vi "FPGA Main.vi"() -> ()   [LabVIEW 2019]
uses:
  Program Files (x86)/National Instruments/LabVIEW 2019/examples/NI SPI IP/R Series/FPGA/Controls/R Series - SPI Master Control Signals.ctl
  <userlib>/_NI SPI IP/FPGA/Controllers/Public/Transfer Settings.ctl
  <vilib>/Platform/TimedLoop/XDataNode/timing_clust.ctl
  <vilib>/Platform/TimedLoop/XDataNode/nitl_modes.ctl
  <vilib>/Platform/TimedLoop/XDataNode/wakeup.ctl
  <userlib>/_NI SPI IP/FPGA/Controllers/Public/Spi Master Inputs.ctl
  <vilib>/rvi/Emulation/niFpgaGetClockAttributes.vi
  <vilib>/rvi/Emulation/niFpgaSctlEmulationGetInTimedLoop.vi
  <vilib>/rvi/Emulation/niFpgaEmulationReportErrorSimple.vi
  <vilib>/rvi/interface/RandomDataEmulation/nirviRandomDataMultiElementFPGAFIFO.vi
  <instcachedir>/0/nirviRandomDataMultiElementFPGAFIFO_1ED88BA00AC641F388A9B1FAA20E354D.lvgen/nirviRandomDataMultiElementFPGAFIFO_1ED88BA00AC641F388A9B1FAA20E354D_002.vi
  <vilib>/rvi/interface/RandomDataEmulation/niFpgaRandomDataHandleErrors.vi
  <vilib>/rvi/Memory/Memory_Emulation/nirvimemoryFastEmulation.vi
  <vilib>/rvi/Memory/Memory_Emulation/nirvimemoryEmulation.vi
  <vilib>/rvi/Emulation/niFpgaEmulationIsFPGAContextNoSignature.vi
  <vilib>/rvi/DataTransferAndStorage/Container/Common/niFpgaContainerGetUniqueNameForEmu.vi
  <vilib>/rvi/Emulation/niFpgaProcessEmulError.vi
  <vilib>/rvi/errors/nirviReportUnexpectedCaseInternalError (U32).vi
  <vilib>/rvi/Emulation/niFpgaCriticalErrorInLSC.vi
  <vilib>/rvi/eio/common/nirviEmuTemplateMethod_errors.vi
  <vilib>/rvi/DataTransferAndStorage/Container/XNode/niFpgaContainer.xnode
  <vilib>/rvi/interface/RandomDataEmulation/nirviRandomDataFpgaMultiElementTemplate.vi
  <vilib>/eio/EIONode/EIONode.xnode
  <vilib>/Platform/TimedLoop/XDataNode/XDataNode.xnode
  <vilib>/rvi/interface/RandomDataEmulation/nirviRandomDataFpgaReadWriteTemplate.vi
  <userlib>/_NI SPI IP/FPGA/Controllers/NI SPI IP FPGA.lvlib
  <vilib>/Platform/TimedLoop/XDataNode/XDNodeRunTimeDep.lvlib
panel:
  in  "Height":i32=320
  in  "Width":i32=480
  in  "StreamDisabled":bool=TRUE
  in  "Master Settings":T1
  out "Master Signals":T2
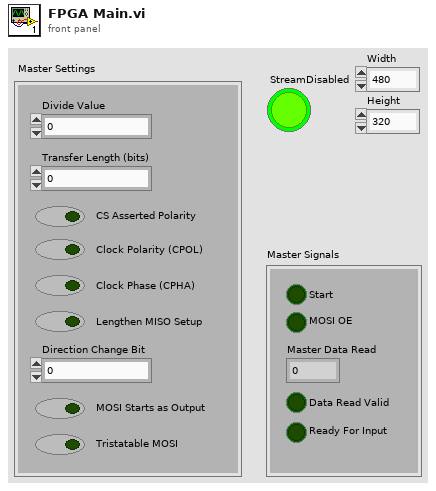
[diagram p1: front panel]
types:
  T1 = typedef "NI SPI IP FPGA.lvlib/Transfer Settings.ctl" = cluster{"Divide Value":u8, "Transfer Length (bits)":u8, "CS Asserted Polarity":bool, "Clock Polarity (CPOL)":bool, "Clock Phase (CPHA)":bool, "Lengthen MISO Setup":bool, "Direction Change Bit":u8, "MOSI Starts as Output":bool, "Tristatable MOSI":bool}
  T2 = typedef "R Series - SPI Master Control Signals.ctl" = cluster{"Start":bool, "MOSI OE":bool, "Master Data Read":u64, "Data Read Valid":bool, "Ready For Input":bool}
  T3 = typedef "XDNodeRunTimeDep.lvlib/timing_clust.ctl" = cluster{"Expected End [f-1]":u64, "Actual End [f-1]":u64, "Finished Late? [f-1]":bool, "Expected End [i-1]":u64, "Actual End [i-1]":u64, "Finished Late? [i-1]":bool, "Expected Start [i]":u64, "Actual Start [i]":u64, "Expected Start [f]":u64, "Actual Start [f]":u64, "Source Name":string, "Structure Name":string, "Period":i64, "Deadline":i64, "Offset":i64, "Start":i64, "Priority":i32, "Timeout":i32, "Mode":T4, "Wakeup Reason":T5, "Error":errorcluster, "Source Type":string, "Secondary Source Type":string, "Global End Time":u64, "Global Start Time":u64, "Frame Duration":u64, "Iteration Duration":u64, "Assigned CPU":i32, "I/O Scan Engine Mode":u32}
  T4 = typedef "XDNodeRunTimeDep.lvlib/nitl_modes.ctl" = enum32{"No Change", "Process missed periods, maintain original phase", "Discard missed periods, maintain original phase", "Process missed periods, ignore original phase", "Discard missed periods, ignore original phase"}
  T5 = typedef "XDNodeRunTimeDep.lvlib/wakeup.ctl" = enum32{"Normal", "Aborted", "Asynchronous wakeup", "Timing source error", "Timed loop error", "Timeout"}
  T6 = typedef "NI SPI IP FPGA.lvlib/Spi Master Inputs.ctl" = cluster{"MISO":bool}
  T7 = typedef "NI SPI IP FPGA.lvlib/Spi Master Outputs.ctl" = cluster{"Chip Select":bool, "Clock":bool, "MOSI":bool, "MOSI OE":bool}
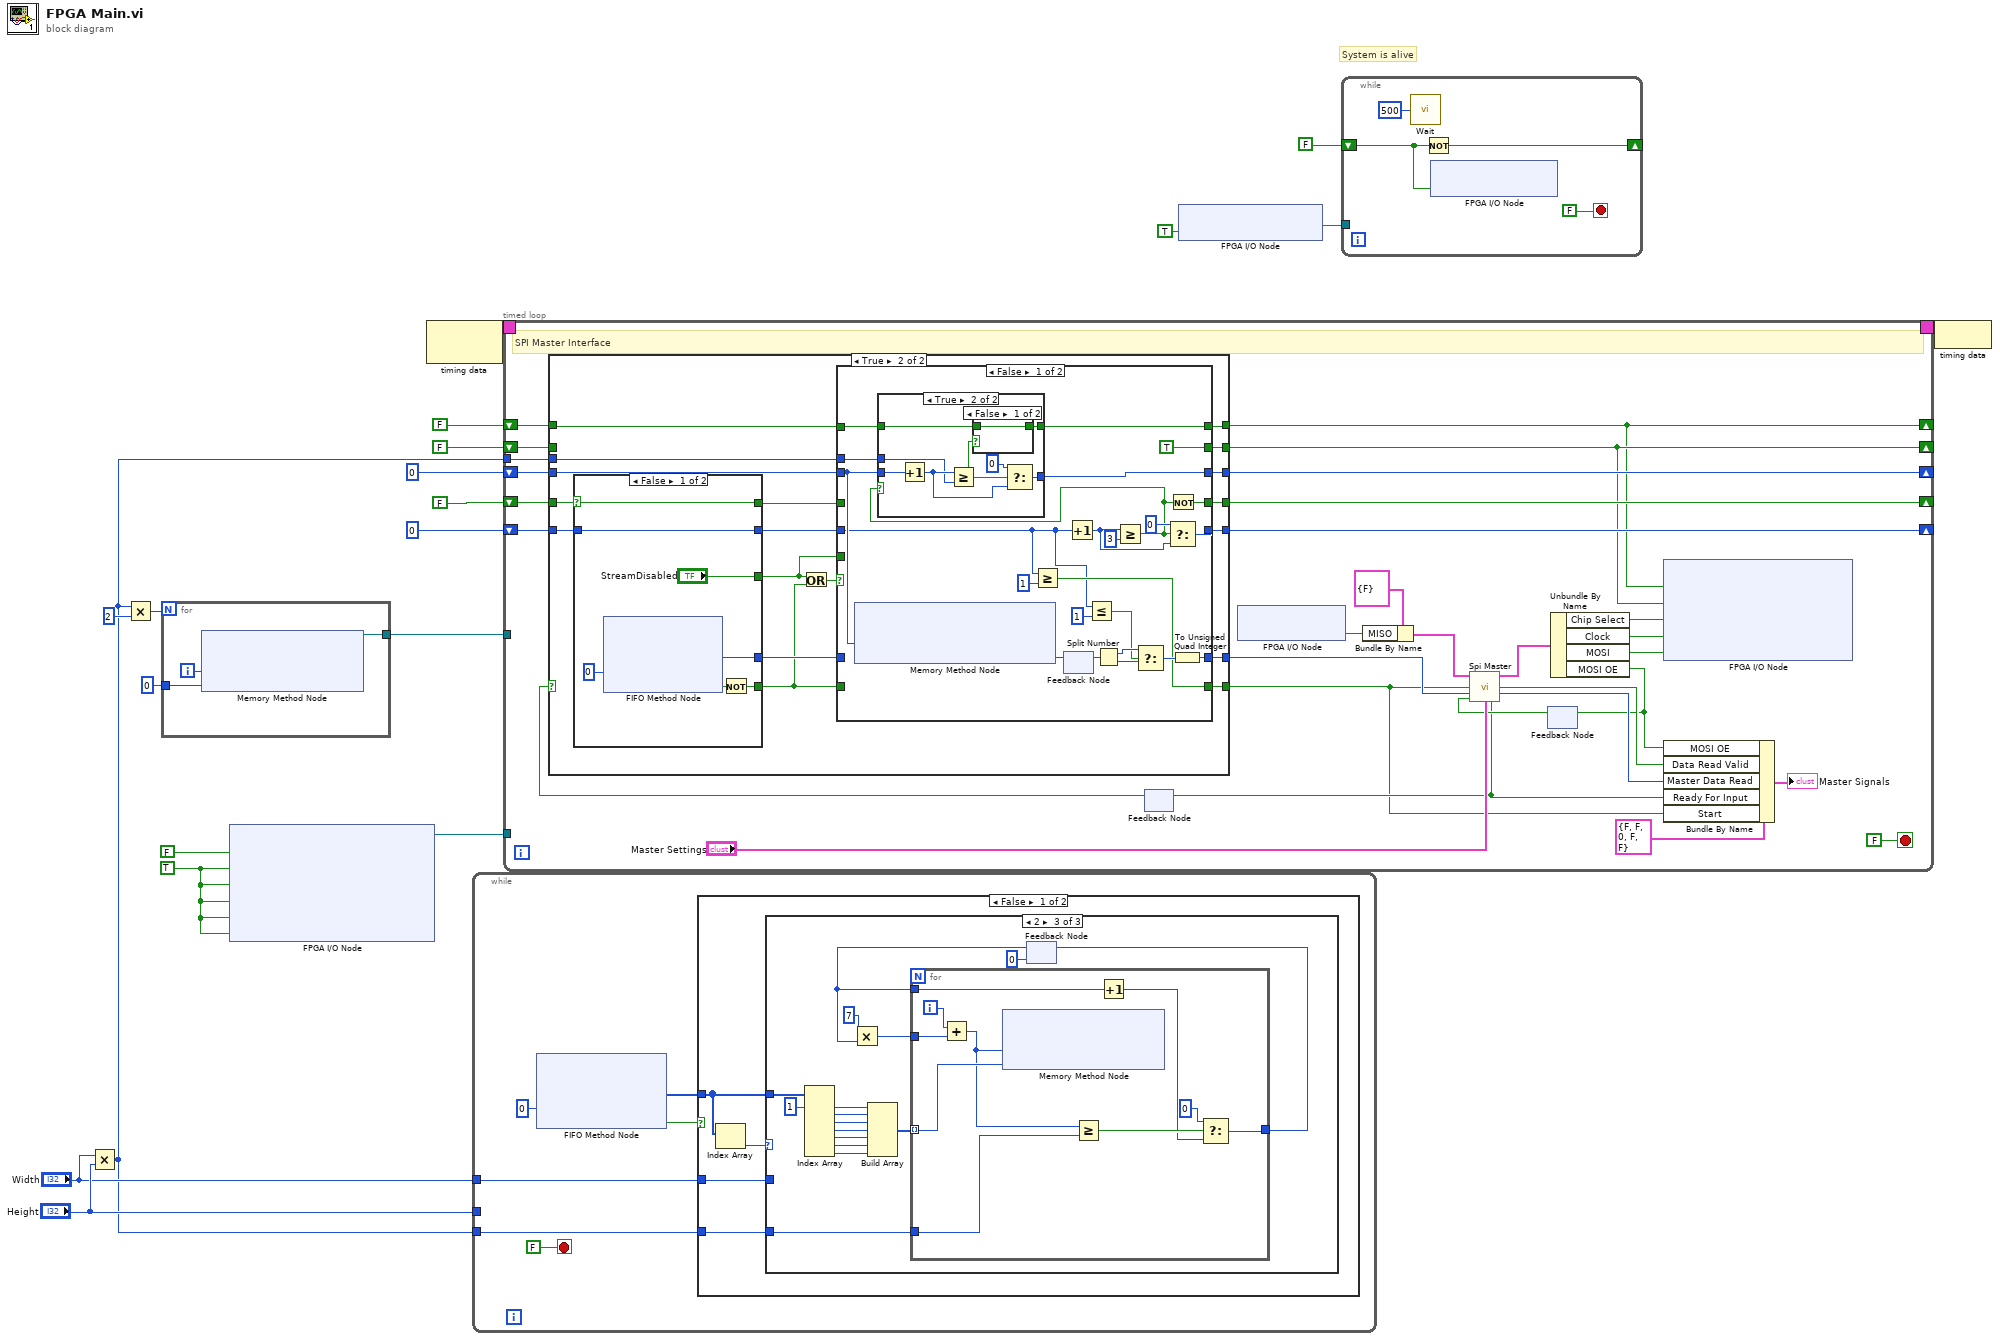
[diagram p0: block diagram]
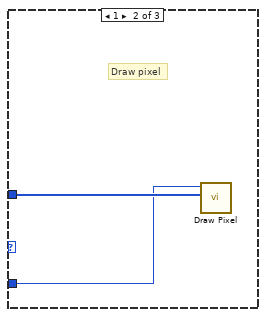
[diagram p3: hidden frame]
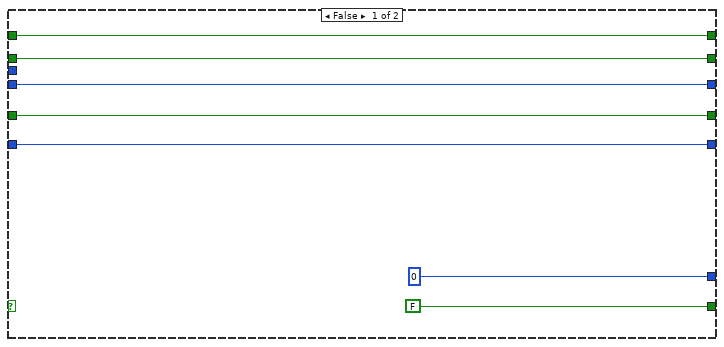
[diagram p5: hidden frame]
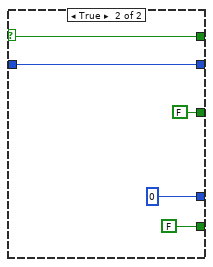
[diagram p6: hidden frame]
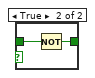
[diagram p8: hidden frame]
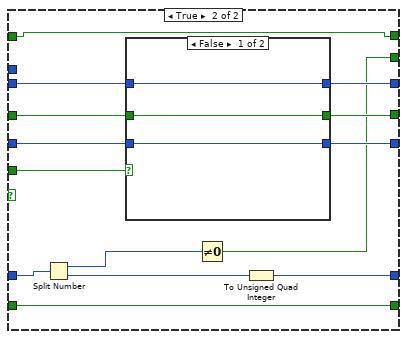
[diagram p9: hidden frame]
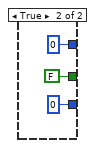
[diagram p10: hidden frame]
diagram:
  w3 = TRUE ("DevKit\\MISO_enable")
  # "System is alive"
  n1 = Multiply(x="Width", y="Height") -> (x*y=w1:i32)
  n2 = Multiply(x=w1, y=2) -> (x*y=w4:i32)
  n3 = for {
    N: w4 -> [_]
    tunnel: 0 -> [w22]
    tunnel: [w21] -> w9
    i -> [w23]
    n4 = xnode ("Memory Method Node")("Address"=w23, "Data"=w22) -> ("Memory Out"=w21:refnum<k21>)  [unwired: 1 in]
  }
  n5 = xnode "FPGA I/O Node"("DevKit\\MISO_enable"=FALSE ("DevKit\\MISO_enable"), "DevKit\\CS_enable"=w3, "DevKit\\CLK_enable"=w3, "DevKit\\MOSI_enable"=w3, "DevKit\\DC_PMOD1_Pin1_enable"=w3, "DevKit\\PMOD1_Pin2_enable"=w3) -> ("FPGA I/O Out"=w14:refnum<k21>)  [unwired: 6 in, 5 out]
  n6 = node-c288() -> (w17:T3)  [unwired: 1 in]
  n7 = while {
    tunnel: "Width" -> [w25]
    tunnel: "Height" -> [_]
    tunnel: w1 -> [w24]
    stop <- FALSE stop-if-true
    n8 = xnode ("FIFO Method Node")("Timeout"=0) -> ("Element"=w27:u16[], "Timed Out?"=w26:bool)  [unwired: 1 in, 1 out]
    n9 = case shown="False" w26 {
      tunnel: w27 -> [w32 _]
      tunnel: w25 -> [w31 _]
      tunnel: w24 -> [w30 _]
      frame False {
        n10 = Index Array(array=w32) -> (element=w33:u16)  [unwired: 1 in]
        n11 = case shown="2" w33 {
          tunnel: w32 -> [_ w35 w50]
          tunnel: w31 -> [_ w34 _]
          tunnel: w30 -> [_ _ w37]
          frame Default {
          }
          frame 1 {
            # "Draw pixel"
            n12 = call "Draw Pixel.vi"("Data"=w35, "Width"=w34) -> ()  [unwired: 10 in]
          }
          frame 2 {
            n13 = Index Array(array=w50, index #1=1 ("index")) -> (element #1=w48:u16, element #2=w47:u16, element #3=w46:u16, element #4=w45:u16, element #5=w44:u16, element #6=w43:u16, element #7=w42:u16)  [unwired: 6 in]
            n14 = Build Array(w48, w47, w46, w45, w44, w43, w42) -> (w41:u16[])
            n15 = feedback #1(u32 0) -> (w38:u32)
            n16 = Multiply(x=u32 7, y=w38) -> (x*y=w40:u32)
            n17 = for {
              tunnel: w41 -> [w59] mode=indexing
              tunnel: w40 -> [w60]
              tunnel: w38 -> [w58]
              tunnel: w37 -> [w56]
              tunnel: [w52] -> w36
              i -> [w61]
              n18 = Add(x=w61, y=w60) -> (x+y=w57:u32)
              n19 = xnode ("Memory Method Node")("Address"=w57, "Data"=w59) -> ()  [unwired: 1 in, 1 out]
              n20 = Greater Or Equal?(x=w57, y=w56) -> (x >= y?=w55:bool)
              n21 = Increment(x=w58) -> (x+1=w53:u32)
              n22 = Select(t=u32 0, s=w55, f=w53) -> (s? t:f=w52:u32)
            }
            n23 = feedback-in #1(w36) -> ()
          }
        }
      }
      frame True {
      }
    }
  }
  n24 = timed-loop "SPI Master Interface" {
    timing: w17 -> [_]
    timing-out: [_] -> w16
    tunnel: w14 -> [_]
    shift-right: [w70] -> _
    shift-left: u8 0 ("Address") -> [w72]
    shift-right: [w69] -> _
    shift-left: 0 ("Address") -> [w71]
    shift-right: [w68] -> _
    shift-left: FALSE ("sbRIO-9651 Socket\\PMOD_I2C_SCL1_enable") -> [w67]
    tunnel: w9 -> [_]
    shift-right: [w65] -> _
    shift-left: FALSE ("sbRIO-9651 Socket\\PMOD_I2C_SCL1_enable") -> [w66]
    tunnel: w1 -> [w64]
    shift-right: [w62] -> _
    shift-left: FALSE ("sbRIO-9651 Socket\\PMOD_I2C_SCL1_enable") -> [w63]
    stop <- FALSE stop-if-true
    # "SPI Master Interface"
    n25 = feedback #2() -> (w74:bool)  [unwired: 1 in]
    n26 = case shown="True" w74 {
      tunnel: [FALSE ("Timed Out?") w116] -> w73
      tunnel: [u64 0 ("Element") w115] -> w76
      tunnel: w72 -> [w95 w108]
      tunnel: w71 -> [w96 w112]
      tunnel: [w95 w111] -> w70
      tunnel: [w96 w110] -> w69
      tunnel: [w94 w109] -> w68
      tunnel: w67 -> [w94 w107]
      tunnel: w66 -> [w93 _]
      tunnel: [w93 w102] -> w65
      tunnel: w64 -> [_ w101]
      tunnel: w63 -> [w92 w100]
      tunnel: [w92 w99] -> w62
      frame False {
      }
      frame True {
        n27 = case shown="False" w107 {
          selector: w107 -> [w118 w126]
          tunnel: [w121 FALSE] -> w104
          tunnel: [w120 u8 0 ("U8")] -> w114
          tunnel: [w119 w127] -> w113
          tunnel: w108 -> [w119 w127]
          tunnel: [w118 w126] -> w106
          tunnel: ["StreamDisabled" FALSE ("StreamData")] -> w103
          frame False {
            n28 = xnode ("FIFO Method Node")("Timeout"=0) -> ("Element"=w120:u16, "Timed Out?"=w122:bool)  [unwired: 1 in, 1 out]
            n29 = Not(x=w122) -> (.not. x?=w121:bool)
          }
          frame True {
          }
        }
        n30 = Or(x=w103, y=w104) -> (x .or. y?=w105:bool)
        n31 = case shown="False" w105 {
          tunnel: [w134 w178] -> w116
          tunnel: [w139 w170] -> w115
          tunnel: w114 -> [_ w169]
          tunnel: w113 -> [w132 w176]
          tunnel: w112 -> [w150 w174]
          tunnel: [w146 w171] -> w111
          tunnel: [w151 w173] -> w110
          tunnel: [w143 w172] -> w109
          tunnel: w106 -> [_ w175]
          tunnel: w104 -> [_ w178]
          tunnel: w103 -> [_ w177]
          tunnel: [TRUE ("sbRIO-9651 Socket\\PMOD_I2C_SCL1_enable") w167] -> w102
          tunnel: w101 -> [w140 _]
          tunnel: w100 -> [w130 w165]
          tunnel: [w129 w165] -> w99
          frame False {
            n32 = xnode ("Memory Method Node")("Address"=w150) -> ("Data"=w149:u16)  [unwired: 1 in, 1 out]
            n33 = Greater Or Equal?(x=w132, y=u8 1) -> (x >= y?=w134:bool)
            n34 = feedback-in #3(w149) -> ()
            n35 = feedback #3() -> (w138:u16)  [unwired: 1 in]
            n36 = Increment(x=w132) -> (x+1=w145:u8)
            n37 = Less Or Equal?(x=w132, y=u8 1) -> (x <= y?=w131:bool)
            n38 = Split Number(x=w138) -> (hi(x)=w136:u8, lo(x)=w137:u8)
            n39 = Greater Or Equal?(x=w145, y=u8 3) -> (x >= y?=w142:bool)
            n40 = case shown="True" w142 {
              tunnel: [w153 w159] -> w151
              tunnel: w150 -> [w153 w158]
              tunnel: w140 -> [_ w157]
              tunnel: w130 -> [w152 w155]
              tunnel: [w152 w154] -> w129
              frame False {
              }
              frame True {
                n41 = Increment(x=w158) -> (x+1=w161:i32)
                n42 = Greater Or Equal?(x=w161, y=w157) -> (x >= y?=w156:bool)
                n43 = case shown="False" w156 {
                  tunnel: w155 -> [w162 w164]
                  tunnel: [w162 w163] -> w154
                  frame False {
                  }
                  frame True {
                    n44 = Not(x=w164) -> (.not. x?=w163:bool)
                  }
                }
                n45 = Select(t=0, s=w156, f=w161) -> (s? t:f=w159:i32)
              }
            }
            n46 = Select(t=w136, s=w131, f=w137) -> (s? t:f=w135:u8)
            n47 = Select(t=u8 0 ("Address"), s=w142, f=w145) -> (s? t:f=w146:u8)
            n48 = Not(x=w142) -> (.not. x?=w143:bool)
            n49 = To Unsigned Quad Integer(1:w135) -> (0:w139:u64)
          }
          frame True {
            n50 = Split Number(x=w169) -> (hi(x)=w166:u8, lo(x)=w168:u8)
            n51 = case shown="False" w177 {
              tunnel: w176 -> [w179 _]
              tunnel: w175 -> [w180 _]
              tunnel: w174 -> [w181 _]
              tunnel: [w181 0 ("Address")] -> w173
              tunnel: [w180 FALSE] -> w172
              tunnel: [w179 u8 0 ("Address")] -> w171
              frame False {
              }
              frame True {
              }
            }
            n52 = Not Equal To 0?(x=w166) -> (x != 0?=w167:bool)
            n53 = To Unsigned Quad Integer(1:w168) -> (0:w170:u64)
          }
        }
      }
    }
    n54 = xnode "FPGA I/O Node"() -> ("DevKit\\MISO"=w77:bool)  [unwired: 1 in, 1 out]
    n55 = Bundle By Name(cluster=T6 {"MISO"=FALSE} ("SPI.Input"), "MISO"=w77) -> (w87:T6)
    n56 = feedback #4() -> (w84:bool)  [unwired: 1 in]
    n57 = call <userlib>:"Spi Master.vi"("spi input"=w87, "start strobe"=w73, "data to write"=w76, "MOSI output enable done"=w84, "spi transfer settings"="Master Settings") -> ("spi output"=w91:T7, "read data valid"=w80:bool, "read data"=w81:u64, "ready for input"=w75:bool)  [unwired: 7 in]
    n58 = feedback-in #2(w75) -> ()
    n59 = Unbundle By Name(w91) -> ("Chip Select"=w88:bool, "Clock"=w90:bool, "MOSI"=w89:bool, "MOSI OE"=w79:bool)
    n60 = feedback-in #4(w79) -> ()
    n61 = xnode "FPGA I/O Node"("DevKit\\PMOD1_Pin2_out"=w62, "DevKit\\DC_PMOD1_Pin1_out"=w65, "DevKit\\CS"=w88, "DevKit\\CLK"=w90, "DevKit\\MOSI"=w89) -> ()  [unwired: 5 in, 5 out]
    n62 = Bundle By Name(cluster=T2 {"Start"=FALSE, "MOSI OE"=FALSE, "Master Data Read"=0, "Data Read Valid"=FALSE, "Ready For Input"=FALSE} ("Master Signals"), "MOSI OE"=w79, "Data Read Valid"=w80, "Master Data Read"=w81, "Ready For Input"=w75, "Start"=w73) -> (→"Master Signals":T2)
  }
  n63 = xnode "FPGA I/O Node"("DevKit\\LED1_enable"=TRUE ("sbRIO-9651 Socket\\PMOD_I2C_SCL1_enable")) -> ("FPGA I/O Out"=w18:refnum<k21>)  [unwired: 1 in]
  n64 = while {
    shift-right: [w190] -> _
    shift-left: FALSE ("sbRIO-9651 Socket\\PMOD_I2C_SCL1_enable") -> [w188]
    tunnel: w18 -> [_]
    stop <- FALSE stop-if-true
    n65 = call "Wait"("Count(mSec)"=u32 500) -> ()  [unwired: 1 out]
    n66 = Not(x=w188) -> (.not. x?=w190:bool)
    n67 = xnode "FPGA I/O Node"("DevKit\\LED1_out"=w188) -> ()  [unwired: 1 in, 1 out]
  }
  n68 = node-c288(w16) -> ()
